vi "GetFlags.vi"(8 "error in (no error)":errorcluster, 11 "IEC61850FlagImpairPlugin in":refnum<class "IEC61850FlagImpairPlugin.lvclass">) -> (0 "error out":errorcluster, 3 "IEC61850FlagImpairPlugin out":refnum<class "IEC61850FlagImpairPlugin.lvclass">)   [LabVIEW 2017, in "FlagImpairPlugins.lvlib" / "IEC61850FlagImpairPlugin.lvclass"]
uses:
  IEC61850FlagImpairPlugin.lvclass
  C:/dev/Work/PARTF/Modules/FlagImpairPlugins/FlagImpairPluginBase_class/FlagImpairPluginBase.lvclass
  FlagImpairPluginBase_class/Accessors/Read clFlagImpairConfig.vi
  FlagImpairPluginBase_class/Accessors/Read FlagImpairParams.vi
  FlagImpairPluginBase_class/Accessors/Read TimeArray.vi
  FlagImpairPluginBase_class/Accessors/Set FlagImpairmentArray.vi
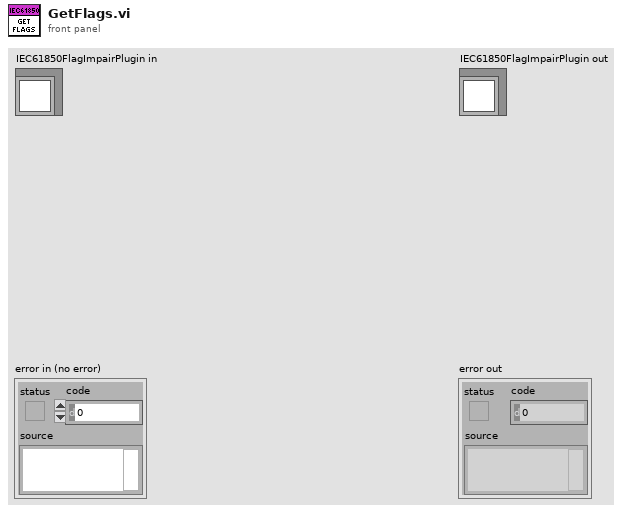
[diagram p1: front panel]
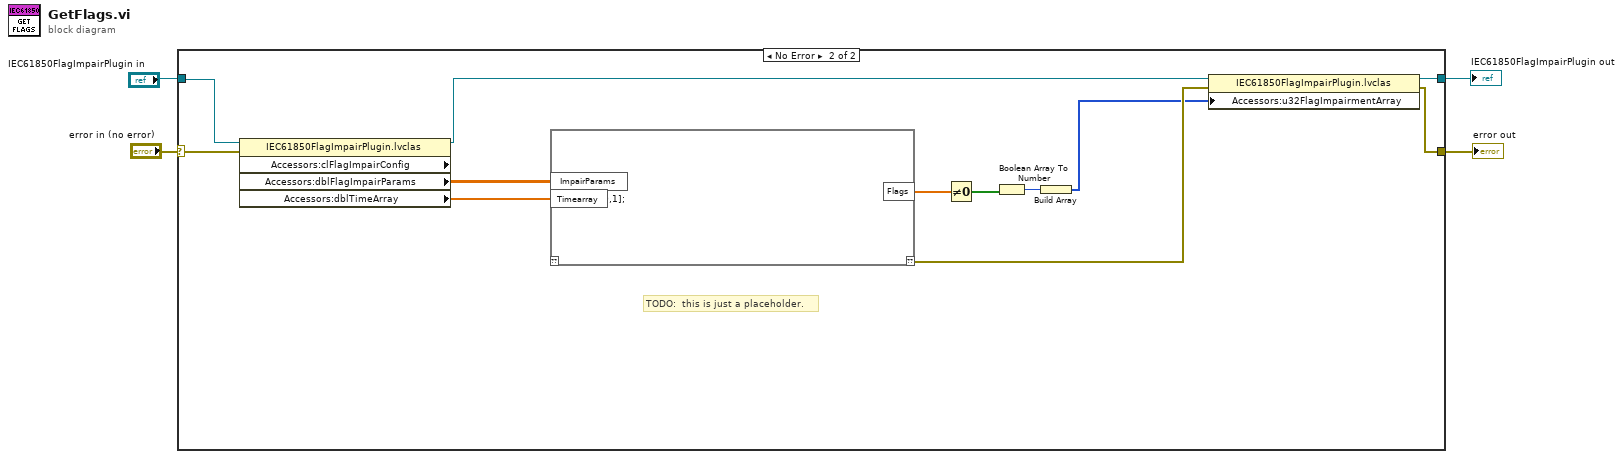
[diagram p0: block diagram]
diagram:
  n1 = case shown="No Error" "error in (no error)" {
    selector: "error in (no error)" -> [w6 w15]
    tunnel: [w5 w18] -> w2
    tunnel: "IEC61850FlagImpairPlugin in" -> [w5 w16]
    tunnel: [w6 w17] -> w1
    frame Error {
    }
    frame No Error {
      # "TODO:  this is just a placeholder."
      n2 = property class="IEC61850FlagImpairPlugin.lvclas" props=["Accessors:clFlagImpairConfig", "Accessors:dblFlagImpairParams", "Accessors:dblTimeArray"](reference=w16, error in=w15) -> (reference out=w14:refnum<class "IEC61850FlagImpairPlugin.lvclass">, "Accessors:dblFlagImpairParams"=w12:dbl[][], "Accessors:dblTimeArray"=w11:dbl[])  [unwired: 2 out]
      n3 = script code="Flags = [0,1];"("ImpairParams"=w12, "Timearray"=w11) -> ("??"=w13:errorcluster, "Flags"=w10:dbl[])  [unwired: 1 in]
      n4 = Not Equal To 0?(x=w10) -> (x != 0?=w9:bool[])
      n5 = Boolean Array To Number(Boolean array=w9) -> (number=w8:u32)
      n6 = Build Array(w8) -> (w7:u32[])
      n7 = property class="IEC61850FlagImpairPlugin.lvclas"(reference=w14, error in=w13, "Accessors:u32FlagImpairmentArray"=w7) -> (reference out=w18:refnum<class "IEC61850FlagImpairPlugin.lvclass">, error out=w17:errorcluster)
    }
  }
  "error out" <- w1
  "IEC61850FlagImpairPlugin out" <- w2
